vi "Datasheet Queue Handler.vi"(0 "Datasheet Queue":refnum<queue>) -> ()   [LabVIEW 2011]
uses:
  Datasheet/Datasheet Inputs.ctl
  www/cgi-bin/_cgi-lib/TDM_INDEX Record.ctl
  Datasheet/Datasheet Generator Settings.ctl
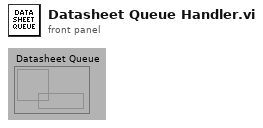
[diagram p1: front panel]
types:
  T1 = typedef "DATASHEET INPUTS.ctl" = cluster{"Items":T2[], "Templates":string[], "Generator Settings":T3, "Response Queue Name":string}
  T2 = typedef "TDM_INDEX Record.ctl" = cluster{"Model Number":string, "SN for sort":i32, "Test Type":string, "Test Run":string, "Serial Number":string, "Start Timestamp":timestamp, "Data File":path, "Result Columns":string[]}
  T3 = typedef "DATASHEET Generator Settings.ctl" = cluster{"Wait? (t)":bool, "ClientPrint? (f)":bool, "Client (\"\")":string, "joinPDF":bool, "Sort Method":enum16{"Item", "Template", "No Sort"}, "Export Row (-1=all)":i32, "Preview":bool, "Estimate Time":bool, "username":string, "jobid":string}
  T4 = typedef "Datasheet Outputs.ctl" = cluster{"Datasheet Paths":T5[], "Actual (Sec)":i32, "error out":errorcluster}
  T5 = typedef "Datasheet Report Info.ctl" = cluster{"sxTemplateId":string[], "reportPath":path}
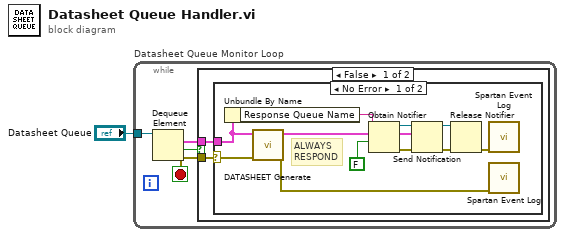
[diagram p0: block diagram]
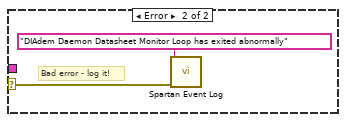
[diagram p2: hidden frame]
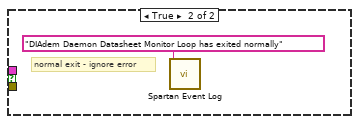
[diagram p3: hidden frame]
diagram:
  n1 = while "Datasheet Queue Monitor Loop" {
    tunnel: "Datasheet Queue" -> [w5]
    stop <- w2 stop-if-true
    n2 = Dequeue Element(queue=w5) -> (element=w4:T1, timed out?=w3:bool, error out=w2:errorcluster)  [unwired: 1 in, 2 out]
    n3 = case shown="False" w3 {
      tunnel: w4 -> [w7 _]
      tunnel: w2 -> [w6 _]
      frame False {
        n4 = case shown="No Error" w6 {
          selector: w6 -> [w18 w19]
          tunnel: w7 -> [w17 _]
          frame No Error {
            # "ALWAYS\nRESPOND"
            n5 = Unbundle By Name(w17) -> ("Response Queue Name"=w8:string)
            n6 = call "DATASHEET Generate.vi"("error in (no error)"=w18, "Datasheet Inputs"=w17) -> ("error out"=w10:errorcluster, "Datasheet Outputs"=w11:T4)  [unwired: 8 in]
            n7 = Obtain Notifier(name (unnamed)=w8, notification data type=w11, create if not found? (T)=FALSE) -> (notifier out=w15:refnum<notifier>, error out=w14:errorcluster)  [unwired: 1 in, 1 out]
            n8 = Send Notification(notification=w11, notifier=w15, error in (no error)=w14) -> (notifier out=w13:refnum<notifier>, error out=w12:errorcluster)
            n9 = Release Notifier(notifier=w13, error in (no error)=w12) -> (error out=w9:errorcluster)  [unwired: 1 in, 2 out]
            n10 = call "Spartan Event Log.vi"("error in (no error)"=w9) -> ()  [unwired: 4 in, 4 out]
            n11 = call "Spartan Event Log.vi"("error in (no error)"=w10) -> ()  [unwired: 4 in, 4 out]
          }
          frame Error {
            # "Bad error - log it!"
            n12 = call "Spartan Event Log.vi"("error in (no error)"=w19, "message (\"\")"="DIAdem Daemon Datasheet Monitor Loop has exited abnormally" ("name (unnamed)")) -> ()  [unwired: 3 in, 4 out]
          }
        }
      }
      frame True {
        # "normal exit - ignore error"
        n13 = call "Spartan Event Log.vi"("message (\"\")"="DIAdem Daemon Datasheet Monitor Loop has exited normally" ("message (\"\")")) -> ()  [unwired: 4 in, 4 out]
      }
    }
  }
